vi "Sequencer.vi"() -> ()   [LabVIEW 2011]
panel:
  out "error out":errorcluster
  in  "error in":errorcluster
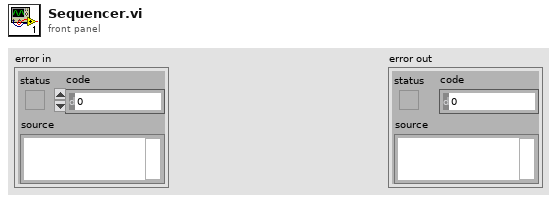
[diagram p1: front panel]
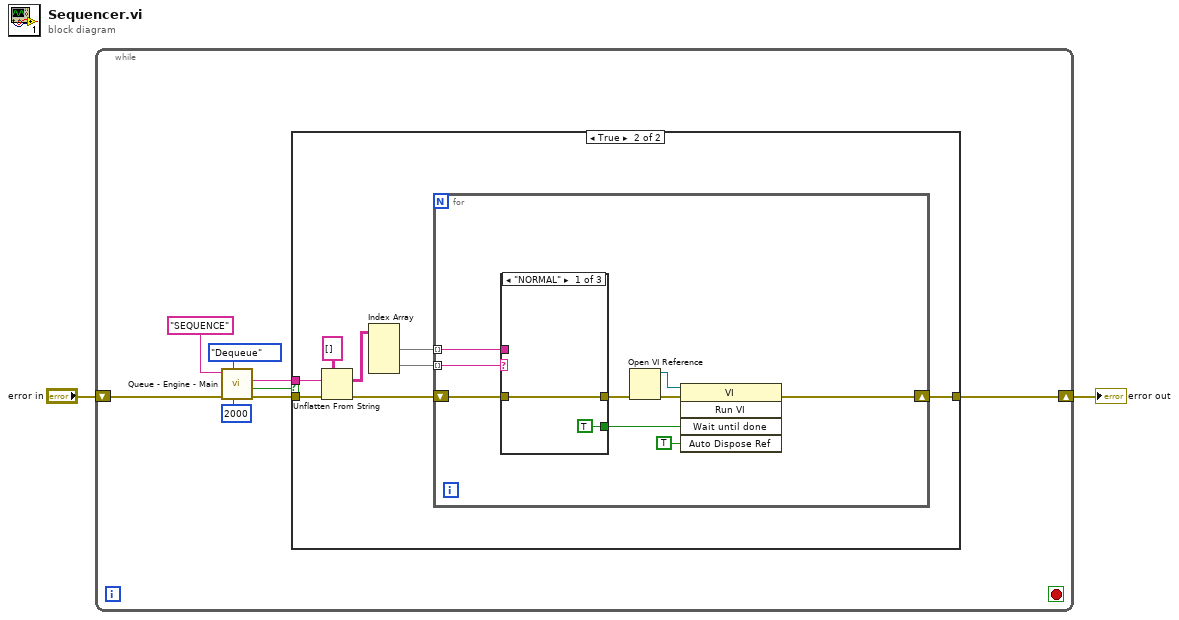
[diagram p0: block diagram]
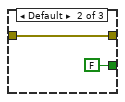
[diagram p3: hidden frame]
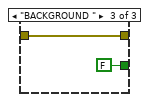
[diagram p4: hidden frame]
diagram:
  n1 = while {
    shift-right: [w4] -> w1
    shift-left: "error in" -> [w7]
    stop <- _ stop-if-true
    n2 = call "Queue - Engine - Main.vi"("timeout in ms (-1)"=2000, "Operation"=enum16{"Enqueue", "Dequeue", "Flush", "Release"}."Dequeue", "error in"=w7, "Queue Name In"="SEQUENCE") -> ("error out"=w8:errorcluster, "timed out?"=w3:bool, "Data Out"=w6:string)  [unwired: 5 in]
    n3 = case shown="True" w3 {
      tunnel: w8 -> [_ w18]
      tunnel: w6 -> [_ w17]
      tunnel: [_ w15] -> w4
      frame False {
      }
      frame True {
        n4 = Unflatten From String(type=string[][] [], binary string=w17, error in (no error)=w18) -> (value=w14:string[][], error out=w16:errorcluster)  [unwired: 2 in, 1 out]
        n5 = Index Array(array=w14) -> (element #1=w13:string[], element #2=w12:string[])  [unwired: 4 in]
        n6 = for {
          shift-right: [w19] -> w15
          shift-left: w16 -> [w26]
          tunnel: w13 -> [w25] mode=indexing
          tunnel: w12 -> [w27] mode=indexing
          n7 = case shown="\"NORMAL\"" w27 {
            tunnel: w26 -> [w29 w30 w32]
            tunnel: w25 -> [_ _ _]
            tunnel: [w29 w30 w32] -> w22
            tunnel: [TRUE ("Wait Until Done") FALSE ("Wait Until Done") FALSE ("Wait Until Done")] -> w24
            frame "NORMAL" {
            }
            frame Default {
            }
            frame "BACKGROUND " {
            }
          }
          n8 = Open VI Reference(error in (no error)=w22) -> (vi reference=w20:refnum<vi>, error out=w21:errorcluster)  [unwired: 5 in]
          n9 = invoke class="VI" method="Run VI"(reference=w20, error in=w21, "Wait until done"=w24, "Auto Dispose Ref"=TRUE ("Auto Dispose Reference")) -> (error out=w19:errorcluster)  [unwired: 1 in, 4 out]
        }
      }
    }
  }
  "error out" <- w1
